vi "tsapp_start_logging.vi"(8 "error in (no error)":errorcluster caption="错误输入（无错误）", 10 "AFullFileName":string, 11 "路径输入":path) -> (0 "error out":errorcluster caption="错误输出", 2 "retuen":i32, 3 "路径输出":path)   [LabVIEW 2014]
doc: "Function Introduction\nStart message recording, record file format is not in BLF format\nCall location\nNeed to record the message communication on the bus throughout the entire operation process\ninput parameter \nAFullFileName: Record the file name (with a suffix of. blf), which can be an empty string\nNote: If AFileName is transmitted as an empty string '', the data file will be stored under the installation path of TSMaster by default.\nThe AFile data format path cannot be incorrect. If the path is invalid, creating the data file will be invalid and trigger internal module errors\nOften.\nReturn value\n==0: Execution successful\nOther values: Query error codes"
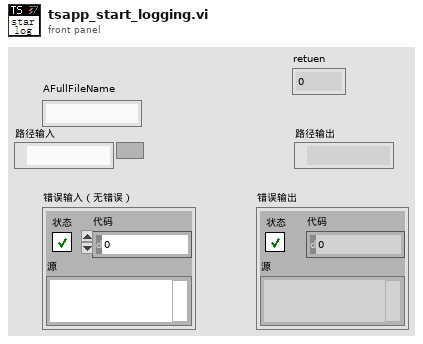
[diagram p1: front panel]
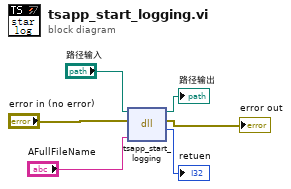
[diagram p0: block diagram]
diagram:
  n1 = dll-call lib="D:/Program Files (x86)/TOSUN/TSMaster/bin/TSMaster.dll" fn="tsapp_start_logging"(path in="路径输入", error in="error in (no error)", "AFullFileName"="AFullFileName") -> (path out=→"路径输出":path, error out=→"error out":errorcluster, "返回类型"=→"retuen":i32)  [unwired: 2 in]
